vi "MaxMinAvg.vi"(3 "Index":i32, 6 "Measurement":fxp<+/-,24,4>) -> (0 "Average Value":sgl, 1 "Minimum Value":fxp<+/-,24,4> format="%.14f", 2 "Maximum Value":fxp<+/-,24,4> format="%.14f")   [LabVIEW 2018]
panel:
  # "Calculate min, max\nand average values.\n\nIf index is 0, it is assumed \nthe first input is received and\nmin, max and averages will be\nset to this value.\n\nOtherwise, it is asusmed next value is received.\nCurrent Min, Max  values are compared with the\nnew value and new average is calculated."
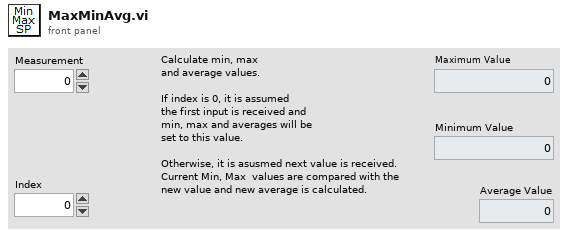
[diagram p1: front panel]
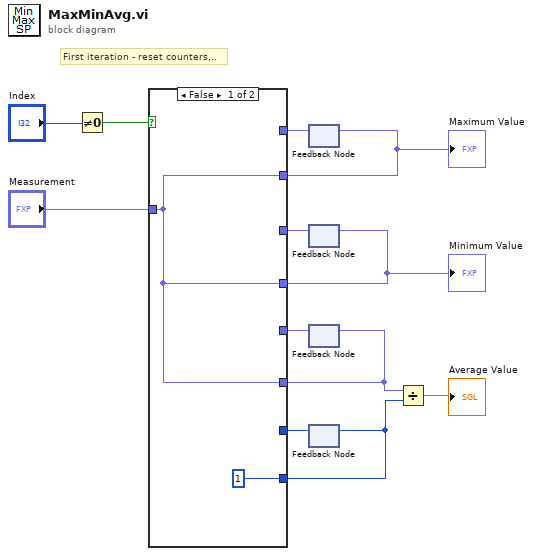
[diagram p0: block diagram]
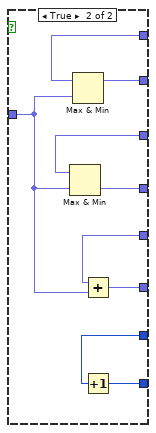
[diagram p2: hidden frame]
diagram:
  # "First iteration - reset counters,.."
  n1 = Not Equal To 0?(x="Index") -> (x != 0?=w9:bool)
  n2 = feedback #1() -> (w11:fxp<+/-,24,4>)  [unwired: 1 in]
  n3 = feedback #2() -> (w7:fxp<+/-,24,4>)  [unwired: 1 in]
  n4 = feedback #3() -> (w2:fxp<+/-,36,16>)  [unwired: 1 in]
  n5 = feedback #4() -> (w3:i32)  [unwired: 1 in]
  n6 = case shown="False" w9 {
    tunnel: [w13 w20] -> w12
    tunnel: "Measurement" -> [w13 w17]
    tunnel: w11 -> [_ w19]
    tunnel: [w13 w18] -> w8
    tunnel: w7 -> [_ w16]
    tunnel: [1 w23] -> w5
    tunnel: [w13 w15] -> w6
    tunnel: w3 -> [_ w22]
    tunnel: w2 -> [_ w21]
    frame False {
    }
    frame True {
      n7 = Max & Min(x=w16, y=w17) -> (min(x,y)=w18:fxp<+/-,24,4>)  [unwired: 1 out]
      n8 = Max & Min(x=w19, y=w17) -> (max(x,y)=w20:fxp<+/-,24,4>)  [unwired: 1 out]
      n9 = Add(x=w21, y=w17) -> (x+y=w15:fxp<+/-,32,16>)
      n10 = Increment(x=w22) -> (x+1=w23:i32)
    }
  }
  "Maximum Value" <- w12
  "Minimum Value" <- w8
  n11 = feedback-in #1(w12) -> ()
  n12 = feedback-in #2(w8) -> ()
  n13 = feedback-in #3(w6) -> ()
  n14 = feedback-in #4(w5) -> ()
  n15 = Divide(x=w6, y=w5) -> (x/y=→"Average Value":sgl)
